vi "Arduino Command Builder.vi"(8 "error in":errorcluster, 10 "Commands":string[](array[string]), 11 "Arduino in":refnum<visa-resource-name>) -> (0 "error out":errorcluster, 3 "Arduino out":refnum<visa-resource-name>)   [LabVIEW 2024]
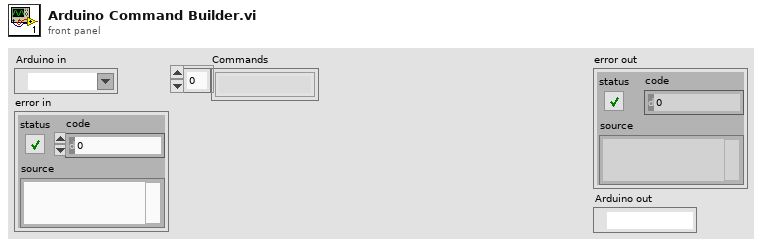
[diagram p1: front panel]
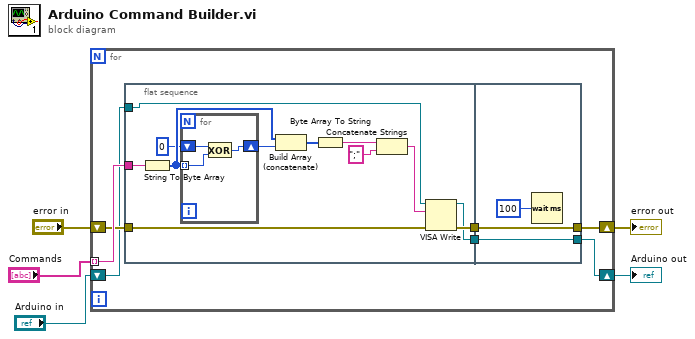
[diagram p0: block diagram]
diagram:
  n1 = for {
    tunnel: "Commands" -> [w12] mode=indexing
    shift-right: [w8] -> w1
    shift-left: "Arduino in" -> [w10]
    shift-right: [w9] -> w2
    shift-left: "error in" -> [w11]
    n2 = flat-sequence {
      tunnel: w12 -> [w24]
      tunnel: w11 -> [w17]
      tunnel: w10 -> [w15]
      tunnel: [w14] -> w7
      tunnel: [w13] -> w6
      tunnel: [w29] -> w8
      tunnel: [w30] -> w9
      tunnel: w7 -> [w30]
      tunnel: w6 -> [w29]
      frame #0 {
        n3 = String To Byte Array(string=w24) -> (unsigned byte array=w21:u8[])
        n4 = for {
          shift-right: [w26] -> w23
          shift-left: u8 0 -> [w27]
          tunnel: w21 -> [w25] mode=indexing
          n5 = Exclusive Or(1:w25, 2:w27) -> (0:w26:u8)
        }
        n6 = Build Array (concatenate)(w21, w23) -> (w22:u8[])
        n7 = Byte Array To String(unsigned byte array=w22) -> (string=w19:string)
        n8 = Concatenate Strings(w19, ";" ("string")) -> (w16:string)
        n9 = VISA Write(VISA resource name=w15, write buffer=w16, error in (no error)=w17) -> (VISA resource name out=w13:refnum<visa-resource-name>, error out=w14:errorcluster)  [unwired: 1 out]
      }
      frame #1 {
        n10 = Wait (ms)(milliseconds to wait=u32 100) -> ()  [unwired: 1 out]
      }
    }
  }
  "error out" <- w2
  "Arduino out" <- w1
